vi "LOC subReadWriteVIStringINIKeys(GraphChart).vi"(4 "Mode":enum16{"Read", "Write"}(ring), 5 "Section":string, 6 "error in (no error)":errorcluster, 8 "ConfigFileRefnum":T1, 9 "ControlRefnum":refnum<vi>) -> (0 "error out":errorcluster)   [LabVIEW 2020, in "Localization_Tools.lvlib"]
uses:
  Localization_Tools.lvlib
  <vilib>/Utility/config.llb/Config Data RefNum.ctl
  <vilib>/Utility/config.llb/NI_LVConfig.lvlib
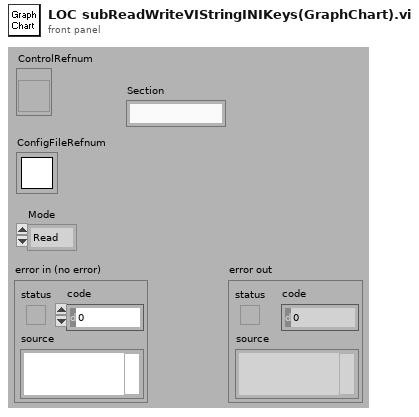
[diagram p1: front panel]
types:
  T1 = typedef "NI_LVConfig.lvlib/Config Data RefNum.ctl" = refnum<k1>
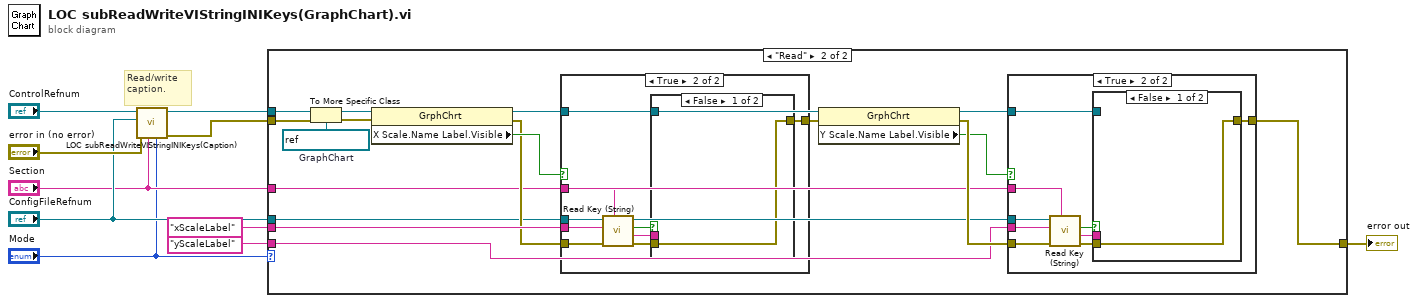
[diagram p0: block diagram]
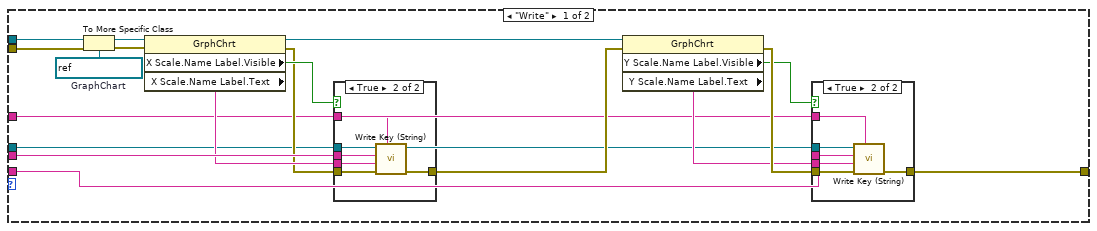
[diagram p2: hidden frame]
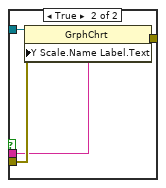
[diagram p6: hidden frame]
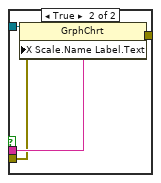
[diagram p8: hidden frame]
diagram:
  # "Read/write\ncaption."
  n1 = call "LOC subReadWriteVIStringINIKeys(Caption).vi"("Mode"="Mode", "Section"="Section", "error in (no error)"="error in (no error)", "ConfigFileRefnum"="ConfigFileRefnum", "ControlRefnum"="ControlRefnum") -> ("error out"=w6:errorcluster, "dup ControlRefnum"=w8:refnum<vi>)  [unwired: 3 in]
  n2 = case shown="\"Read\"" "Mode" {
    tunnel: w8 -> [w27 w58]
    tunnel: w6 -> [w26 w57]
    tunnel: "ConfigFileRefnum" -> [w13 w47]
    tunnel: "Section" -> [w14 w48]
    tunnel: "xScaleLabel" ("key") -> [w23 w54]
    tunnel: [w11 w43] -> w2
    tunnel: "yScaleLabel" ("key") -> [w12 w46]
    frame "Write" {
      w28 = refnum<vi> refnum  # GraphChart
      n3 = To More Specific Class(target class=w28, reference=w27, error in=w26) -> (specific class reference=w25:refnum<vi>, error out=w24:errorcluster)
      n4 = property class="GrphChrt"(reference=w25, error in=w24) -> (reference out=w16:refnum<vi>, error out=w20:errorcluster, "X Scale.Name Label.Visible"=w22:bool, "X Scale.Name Label.Text"=w21:string)
      n5 = case shown="True" w22 {
        tunnel: w13 -> [_ w42]
        tunnel: w14 -> [_ w41]
        tunnel: w23 -> [_ w40]
        tunnel: w21 -> [_ w39]
        tunnel: w20 -> [w36 w38]
        tunnel: [w36 w37] -> w15
        frame False {
        }
        frame True {
          n6 = call <vilib>:"Write Key (String).vi"("section"=w41, "error in (no error)"=w38, "value"=w39, "key"=w40, "refnum"=w42) -> ("error out"=w37:errorcluster)  [unwired: 4 in, 2 out]
        }
      }
      n7 = property class="GrphChrt"(reference=w16, error in=w15) -> (error out=w19:errorcluster, "Y Scale.Name Label.Visible"=w17:bool, "Y Scale.Name Label.Text"=w18:string)  [unwired: 1 out]
      n8 = case shown="True" w17 {
        tunnel: w13 -> [_ w35]
        tunnel: w14 -> [_ w34]
        tunnel: w12 -> [_ w33]
        tunnel: w18 -> [_ w32]
        tunnel: w19 -> [w29 w31]
        tunnel: [w29 w30] -> w11
        frame False {
        }
        frame True {
          n9 = call <vilib>:"Write Key (String).vi"("section"=w34, "error in (no error)"=w31, "value"=w32, "key"=w33, "refnum"=w35) -> ("error out"=w30:errorcluster)  [unwired: 4 in, 2 out]
        }
      }
    }
    frame "Read" {
      w59 = refnum<vi> refnum  # GraphChart
      n10 = To More Specific Class(target class=w59, reference=w58, error in=w57) -> (specific class reference=w56:refnum<vi>, error out=w55:errorcluster)
      n11 = property class="GrphChrt"(reference=w56, error in=w55) -> (reference out=w45:refnum<vi>, error out=w52:errorcluster, "X Scale.Name Label.Visible"=w53:bool)
      n12 = case shown="True" w53 {
        tunnel: w47 -> [_ w84]
        tunnel: w48 -> [_ w83]
        tunnel: w54 -> [_ w82]
        tunnel: w52 -> [w75 w81]
        tunnel: [w75 w77] -> w49
        tunnel: w45 -> [_ w80]
        frame False {
          # "Label not visible, so do nothing"
        }
        frame True {
          n13 = call <vilib>:"Read Key (String).vi"("section"=w83, "error in (no error)"=w81, "key"=w82, "refnum"=w84) -> ("error out"=w78:errorcluster, "value"=w79:string, "found?"=w76:bool)  [unwired: 4 in, 1 out]
          n14 = case shown="False" w76 {
            tunnel: w80 -> [_ w89]
            tunnel: w79 -> [_ w88]
            tunnel: w78 -> [w85 w87]
            tunnel: [w85 w86] -> w77
            frame False {
            }
            frame True {
              n15 = property class="GrphChrt"(reference=w89, error in=w87, "X Scale.Name Label.Text"=w88) -> (error out=w86:errorcluster)  [unwired: 1 out]
            }
          }
        }
      }
      n16 = property class="GrphChrt"(reference=w45, error in=w49) -> (reference out=w44:refnum<vi>, error out=w51:errorcluster, "Y Scale.Name Label.Visible"=w50:bool)
      n17 = case shown="True" w50 {
        tunnel: w47 -> [_ w69]
        tunnel: w48 -> [_ w68]
        tunnel: w46 -> [_ w67]
        tunnel: w51 -> [w60 w66]
        tunnel: w44 -> [_ w65]
        tunnel: [w60 w63] -> w43
        frame False {
          # "Label not visible, so do nothing"
        }
        frame True {
          n18 = call <vilib>:"Read Key (String).vi"("section"=w68, "error in (no error)"=w66, "key"=w67, "refnum"=w69) -> ("error out"=w64:errorcluster, "value"=w62:string, "found?"=w61:bool)  [unwired: 4 in, 1 out]
          n19 = case shown="False" w61 {
            tunnel: w65 -> [_ w74]
            tunnel: w64 -> [w70 w73]
            tunnel: [w70 w72] -> w63
            tunnel: w62 -> [_ w71]
            frame False {
            }
            frame True {
              n20 = property class="GrphChrt"(reference=w74, error in=w73, "Y Scale.Name Label.Text"=w71) -> (error out=w72:errorcluster)  [unwired: 1 out]
            }
          }
        }
      }
    }
  }
  "error out" <- w2
